vi "Software Update HCC Main Update HCC Software.vi"() -> ()   [LabVIEW 2016]
uses:
  Type Definitions/ViperHawk/ViperHawk Diagnostic Data.ctl
panel:
  in  "Update Files (Option 1-24)":i32[](array[numeric])
  in  "Tab Control 2":enum32{"Select Rows", "Find Active Stations"}(tab)
  out "% Complete":u8(slide) scale=0.0..100.0
  in  "Newfi":bool
  in  "Station 4":bool
  in  "Station 3":bool
  in  "Station 2":bool
  in  "Station 1":bool
  in  "Station 5":bool
  in  "Station 6":bool
  in  "Station 7":bool
  in  "Station 8":bool
  in  "Station 9":bool
  in  "Station 10":bool
  in  "Station 11":bool
  in  "Station 12":bool
  in  "Station 13":bool
  in  "Station 14":bool
  in  "Station 15":bool
  in  "Station 16":bool
  in  "Station 17":bool
  in  "Station 18":bool
  in  "Station 19":bool
  in  "Station 20":bool
  in  "Station 21":bool
  in  "Station 22":bool
  in  "Station 23":bool
  in  "Station 24":bool
  in  "Select All 1-4":bool caption="Select Row"
  in  "Select All 5-8":bool caption="Select Row"
  in  "Select All 9-12":bool caption="Select Row"
  in  "Select All 13-16":bool caption="Select Row"
  in  "Select All 17-20":bool caption="Select Row"
  in  "Select All 21-24":bool caption="Select Row"
  in  "Select All":bool
  out "Status String":string
  in  "New Software Location":path
  out "Debug Array":string[](array[string])
  in  "Debug":bool
  out "Main Directory":path
  in  "Find Active Stations":bool
  out "Active Stations with Board IDs":string[][](array[string])
  out "Board ID's":string[](array[string])
  out "Number of Newfi's":i32
  in  "Path Build List":path[](array[path])
  # "Software Update Tool"
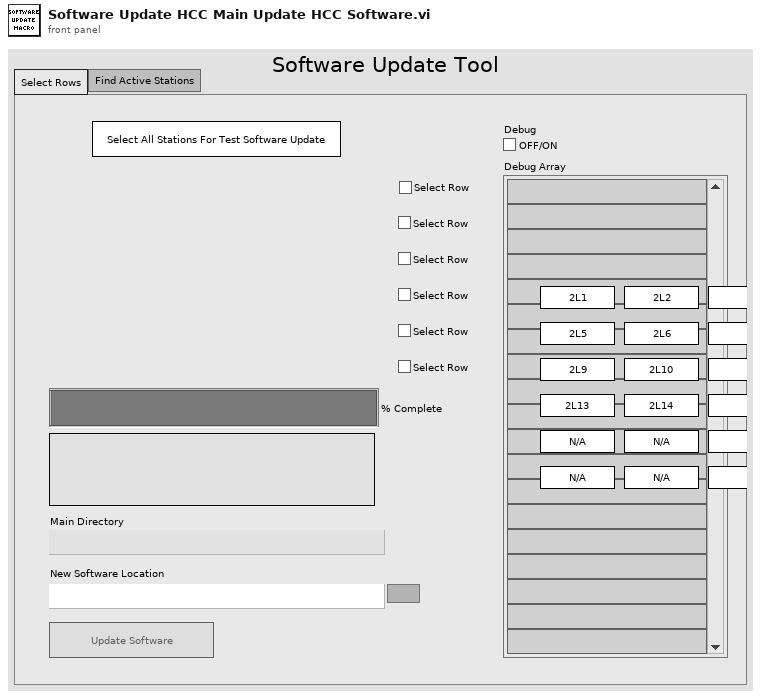
[diagram p1: front panel]
types:
  T1 = enum8{"Enabled", "Disabled", "Disabled and Grayed Out"}
  T2 = enum32{"invalid app kind", "Development System", "Run Time System", "Student Edition", "Embedded LabVIEW", "Evaluation", "Custom"}
  T3 = typedef "ViperHawk Diagnostic Data.ctl" = cluster{"Speed (RPM)":u32, "Load Size":u32, "Temperature":u32, "Water Pressure":dbl, "Detergent":u32, "Fabric Softener":u32, "Tub Direction":string, "Detergent Valve":bool, "Fabric Softener Valve":bool, "Recirculating Pump":bool, "Drain Valve":bool, "Hot Valve":bool, "Cold Valve":bool, "Lid Closed Status":string, "Lid Lock Status":string, "Error Count":u32, "IGBT Temperature (Deg C)":u32, "Motor Speed":u32, "Latched OOB":u32, "Raw OOB":u32, "Plaster Status":u32, "Inverter Power (W)":u32, "Target Speed(BRPM)":u32, "Latched Agitate Motor Temp (Deg C)":u32, "Current Motor Temp (Deg C)":u32, "Profiler Status":string, "Current Inverter Action":string, "Error Codes":string, "Lid Locked":bool, "Lid Closed":bool, "9E Diagnostic Data":cluster{"Total Cycle Time (Min)":u32, "Total Cycle Count (Current)":u16, "Total Error Count":u16, "Machine Error History":u32, "Washer UI History":u32, "Inverter Error History":u32, "Cycle Storage Limit":u8, "Error Storage Limit":u8, "Cycle Pages Supported":u8, "Error Pages Supported":u8, "Inverter Reset Count":u16}, "9F Diagnostic Data":cluster{"Cycle Buffer Index":string, "Page Number":string, "Total Cycle Count":u32, "Delay Start Time":u32, "Stain Selected":string, "Selected Cycle":u32, "eWash":string, "Soil Level":string, "Temperature":string, "Overnight Ready":string, "Spin Setting":string, "Control Lock Status":string, "Stain Remover":string, "Steam Assist":string, "My Cycle":string, "PreWash":string, "Debug Log Enabled":string, "Rinse":string, "Signal Level":string, "PreSoak":string}}
  T4 = enum32{"Invalid", "Standard", "Closed", "Hidden", "Minimized", "Maximized"}
  T5 = cluster{"Core":cluster{"Current VI Reference":refnum<vi>, "Close Panel on Exit?":bool}, "Base Newfi Exe Folder Path":path, "Path Build List":path[], "Update Files (Option 1-24)":i32[], "Diagnostic":T3}
  T6 = cluster{"Current VI Reference":refnum<vi>, "Close Panel on Exit?":bool}
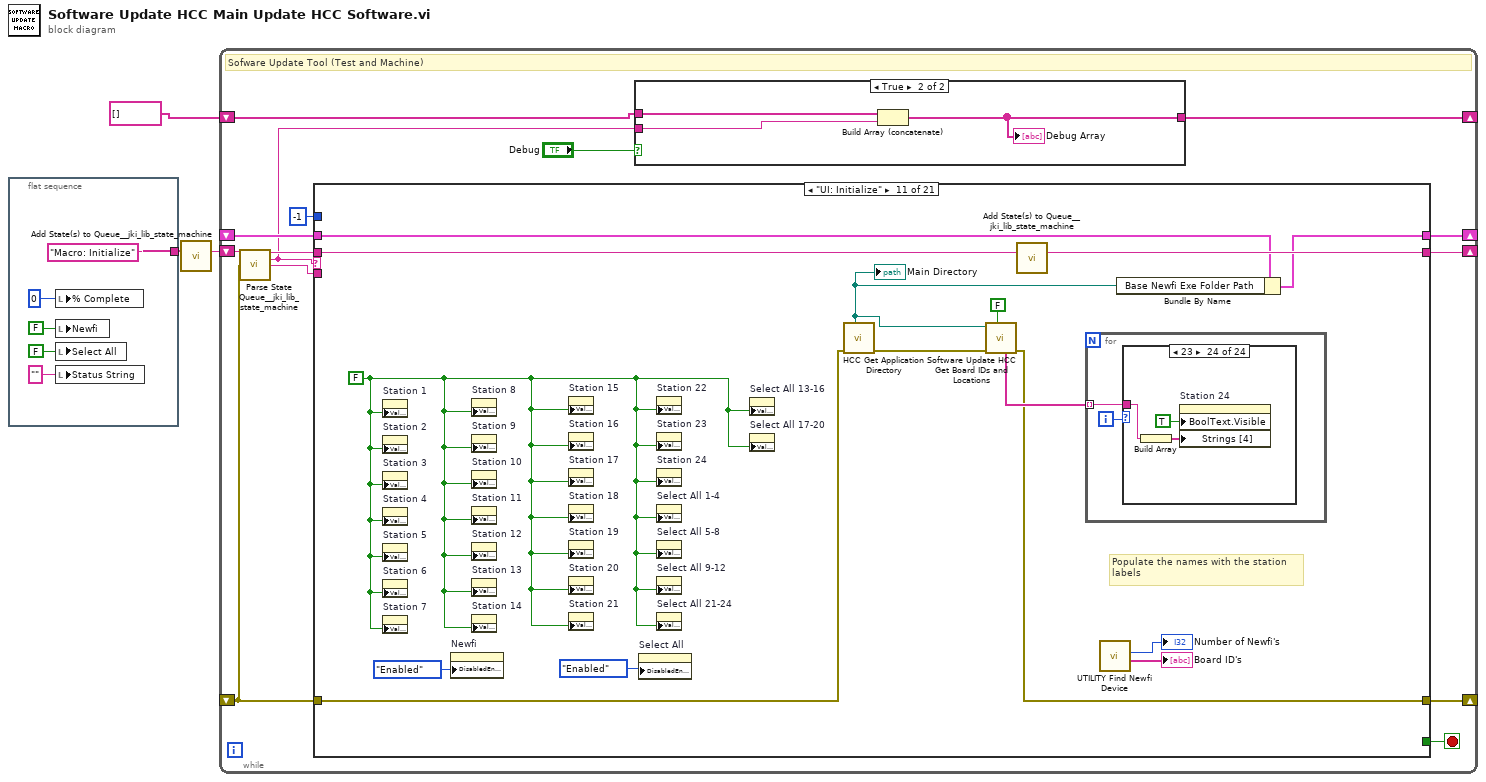
[diagram p0: block diagram]
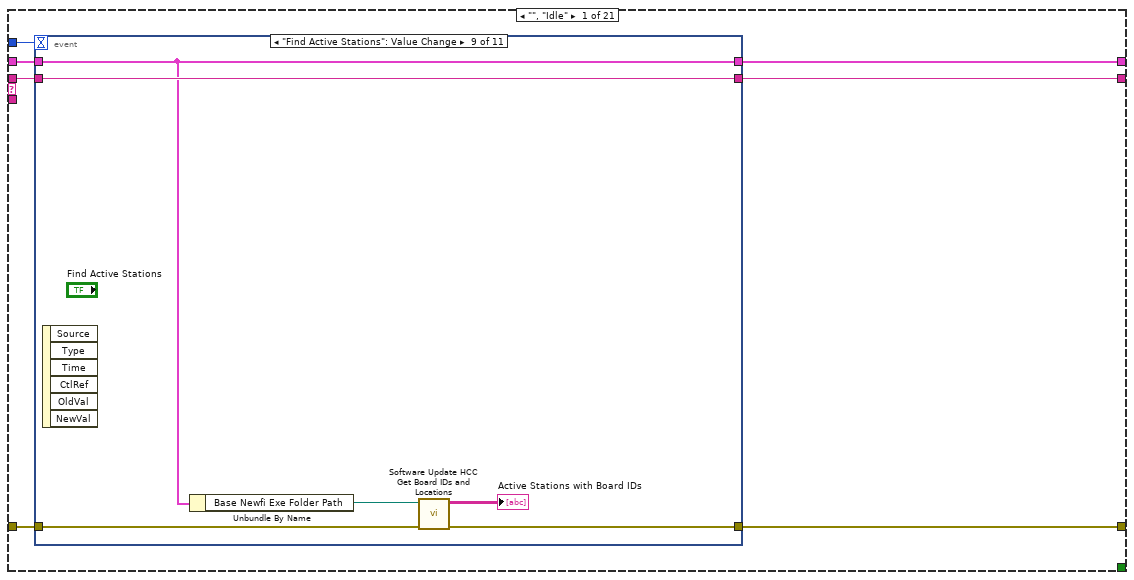
[diagram p3: hidden frame]
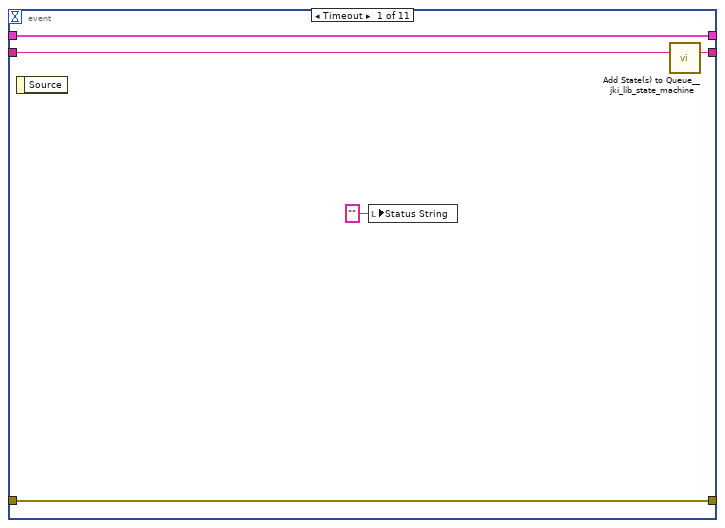
[diagram p4: hidden frame]
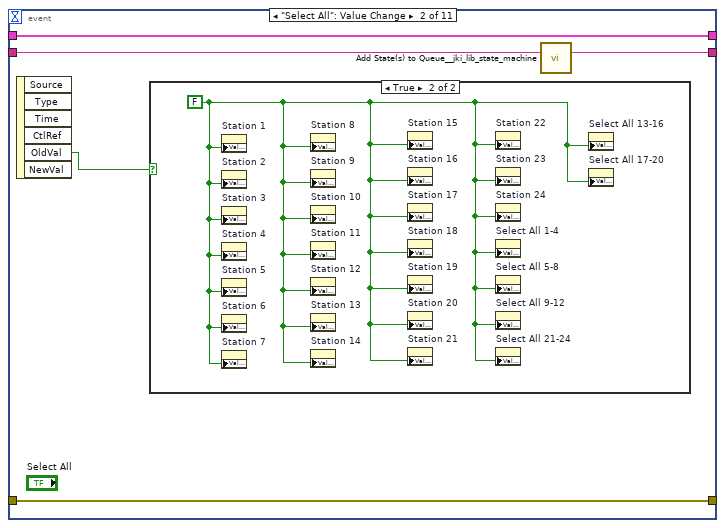
[diagram p5: hidden frame]
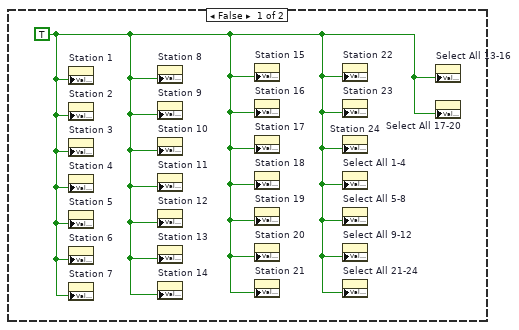
[diagram p6: hidden frame]
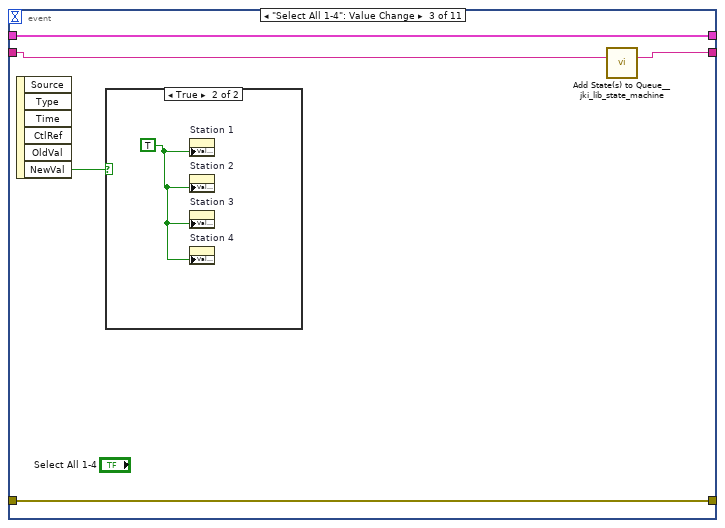
[diagram p7: hidden frame]
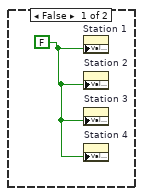
[diagram p8: hidden frame]
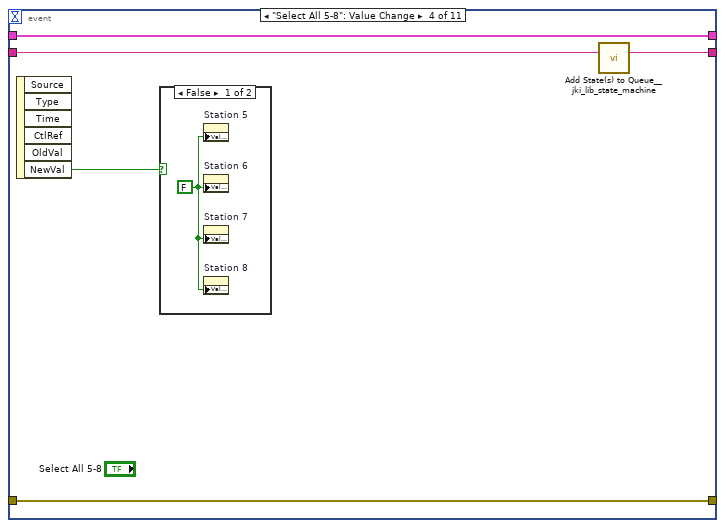
[diagram p9: hidden frame]
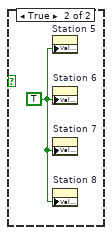
[diagram p10: hidden frame]
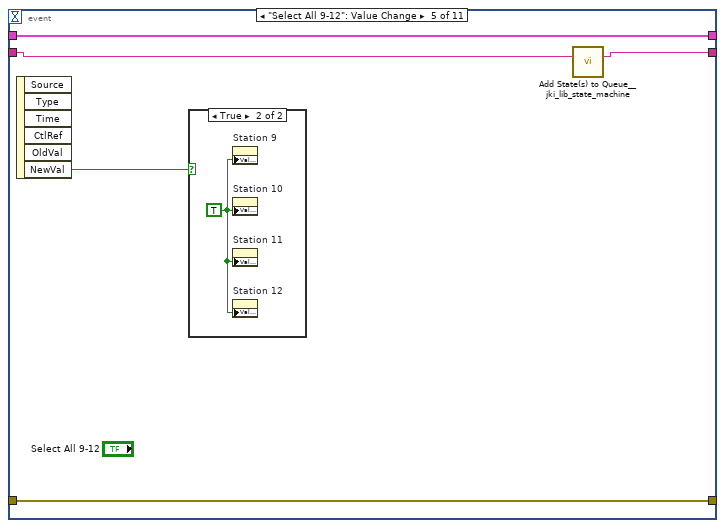
[diagram p11: hidden frame]
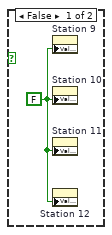
[diagram p12: hidden frame]
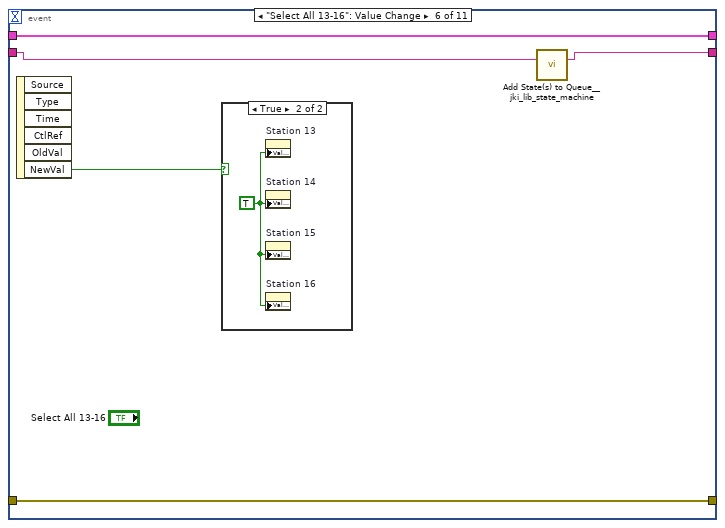
[diagram p13: hidden frame]
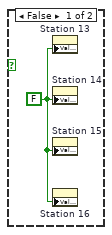
[diagram p14: hidden frame]
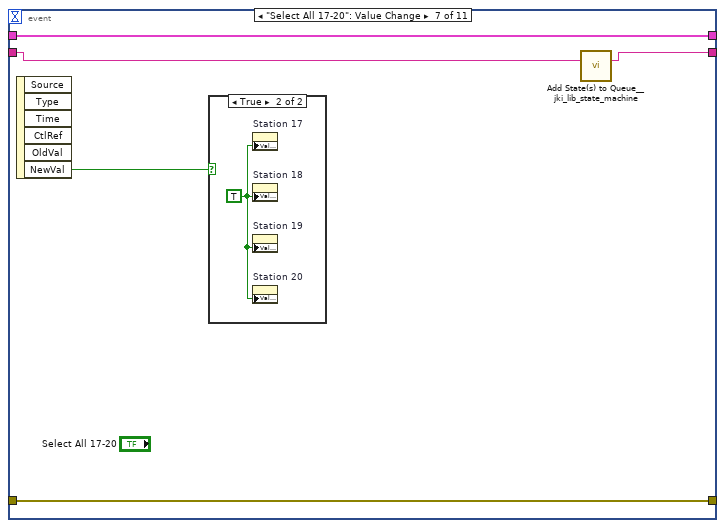
[diagram p15: hidden frame]
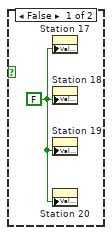
[diagram p16: hidden frame]
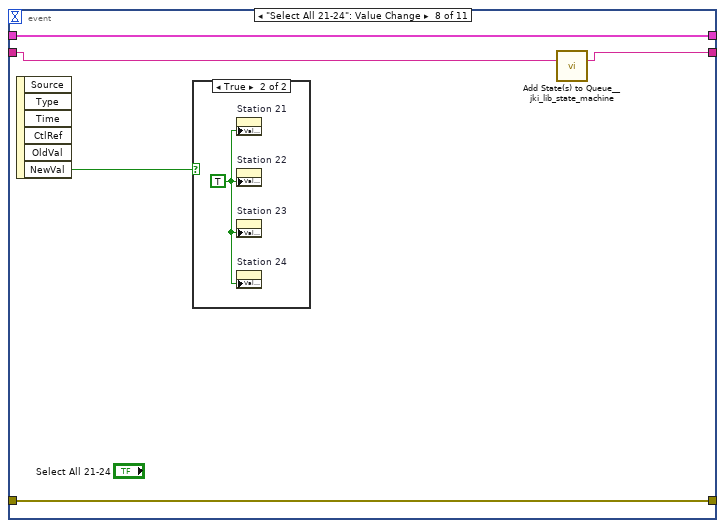
[diagram p17: hidden frame]
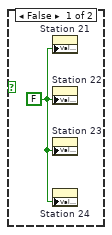
[diagram p18: hidden frame]
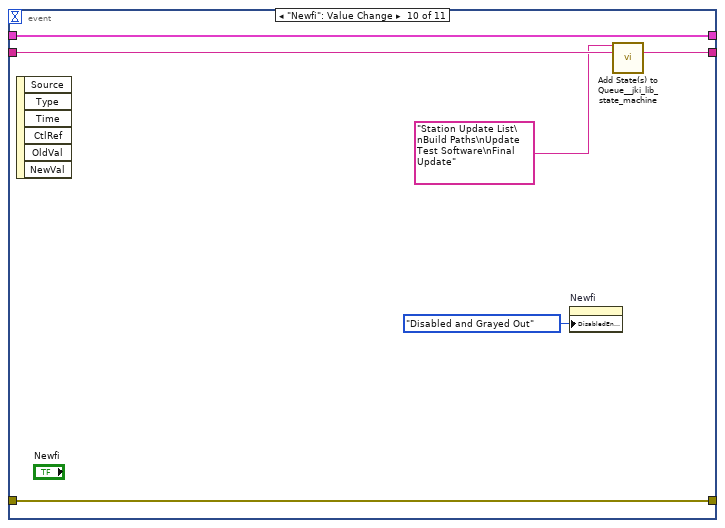
[diagram p19: hidden frame]
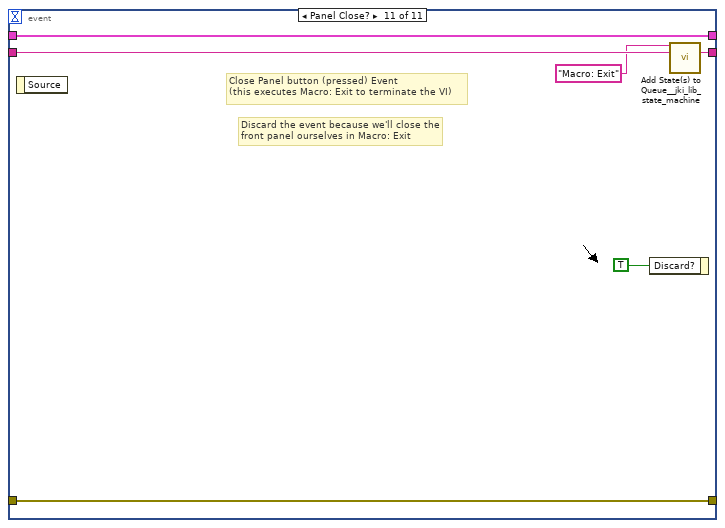
[diagram p20: hidden frame]
diagram:
  n1 = flat-sequence {
    tunnel: ["Macro: Initialize"] -> w2
    frame #0 {
      n2 = local write "% Complete"(u8 0 ("% Complete")) -> ()
      n3 = local write "Newfi"(FALSE ("Newfi")) -> ()
      n4 = local write "Select All"(FALSE ("Select All")) -> ()
      n5 = local write "Status String"("" ("Status String")) -> ()
    }
  }
  n6 = call <vilib>:"Add State(s) to Queue__jki_lib_state_machine.vi"("State(s) in (\"\")"=w2) -> ("States Out"=w3:string)  [unwired: 14 in]
  n7 = while "Sofware Update Tool (Test and Machine)" {
    shift-right: [w16] -> _
    shift-left: _ -> [w15]
    shift-right: [w19] -> _
    shift-left: _ -> [w13]
    shift-right: [w18] -> _
    shift-left: w3 -> [w20]
    shift-right: [w9] -> _
    shift-left: string[] [] -> [w12]
    stop <- w17 stop-if-true
    # "Sofware Update Tool (Test and Machine)"
    n8 = call <vilib>:"Parse State Queue__jki_lib_state_machine.vi"("State Queue"=w20, "Error In (no error)"=w13) -> ("Remaining States"=w22:string, "Current State"=w10:string, "Arguments"=w21:string)  [unwired: 11 in]
    n9 = case shown="\"UI: Initialize\"" w10 {
      selector: w10 -> [_ _ w110 _ _ _ _ _ _ _ _ _ _ _ _ _ _ _ _ _ _]
      tunnel: w22 -> [w33 w109 w114 w132 w138 w143 w147 w156 w162 w166 w181 w261 w272 w298 w303 w314 w318 w353 w363 w378 w386]
      tunnel: w21 -> [_ _ _ _ _ _ _ _ _ _ _ w256 w266 _ _ _ _ _ _ _ _]
      tunnel: w15 -> [w31 w106 w112 w123 w135 w141 w144 _ w157 w163 w169 w259 w268 w295 w300 w311 w315 w350 w360 w374 w384]
      tunnel: [w30 w107 w116 w129 errorcluster {"status"=FALSE, "code"=0, "source"=""} ("error out") w140 w145 w153 w158 w164 w170 w257 w269 w296 w301 w312 w316 w319 w356 w364 w383] -> w19
      tunnel: w13 -> [w29 w107 w115 w129 w134 w140 w145 w153 w159 w164 w171 w258 w270 w296 w301 w312 w316 w320 w357 w365 w383]
      tunnel: [w32 w108 w113 w131 w137 w142 w146 w155 w161 w165 w180 w260 w271 w297 w302 w313 w317 w352 w362 w377 w385] -> w18
      tunnel: [_ _ _ _ _ TRUE _ _ _ _ _ _ _ _ _ _ _ _ _ _ _] -> w17
      tunnel: [w28 w106 w112 w130 w135 w141 w144 w154 w157 w163 w168 w259 w268 w295 w300 w311 w315 w349 w359 w374 w384] -> w16
      tunnel: -1 ("Timeout") -> [w27 _ _ _ _ _ _ _ _ _ _ _ _ _ _ _ _ _ _ _ _]
      frame "", "Idle" {
        n10 = event shown="[8] \"Find Active Stations\": Value Change" {
          selector: _ -> [_ _ _ _ _ _ _ _ _ _ _]
          dyn-events: _ -> [_ _ _ _ _ _ _ _ _ _ _]
          timeout: w27 -> [_ _ _ _ _ _ _ _ _ _ _]
          tunnel: w33 -> [w38 w41 w48 w56 w63 w70 w77 w84 w90 w99 w105]
          tunnel: [w37 w40 w47 w55 w62 w69 w76 w83 w90 w98 w104] -> w32
          tunnel: w31 -> [w35 w43 w49 w57 w64 w71 w78 w85 w89 w94 w102]
          tunnel: [w36 w42 w50 w54 w61 w68 w75 w82 w91 w95 w103] -> w30
          tunnel: w29 -> [w36 w42 w50 w54 w61 w68 w75 w82 w92 w95 w103]
          tunnel: [w35 w43 w49 w57 w64 w71 w78 w85 w89 w94 w102] -> w28
          event Timeout {
            n11 = event-data() -> ()  [unwired: 1 in, 1 out]
            n12 = local write "Status String"("" ("Status String")) -> ()
            n13 = call <vilib>:"Add State(s) to Queue__jki_lib_state_machine.vi"("State(s) in (\"\")"=w38) -> ("States Out"=w37:string)  [unwired: 14 in]
          }
          event "Select All": Value Change {
            n14 = event-data() -> ("OldVal"=w39:bool)  [unwired: 1 in, 5 out]
            n15 = case shown="True" w39 {
              frame False {
                w44 = TRUE
                n16 = property on="Station 1" class="Bool (strict)"("Value"=w44) -> ()  [unwired: 2 in, 2 out]
                n17 = property on="Station 2" class="Bool (strict)"("Value"=w44) -> ()  [unwired: 2 in, 2 out]
                n18 = property on="Station 3" class="Bool (strict)"("Value"=w44) -> ()  [unwired: 2 in, 2 out]
                n19 = property on="Station 4" class="Bool (strict)"("Value"=w44) -> ()  [unwired: 2 in, 2 out]
                n20 = property on="Station 5" class="Bool (strict)"("Value"=w44) -> ()  [unwired: 2 in, 2 out]
                n21 = property on="Station 6" class="Bool (strict)"("Value"=w44) -> ()  [unwired: 2 in, 2 out]
                n22 = property on="Station 7" class="Bool (strict)"("Value"=w44) -> ()  [unwired: 2 in, 2 out]
                n23 = property on="Station 8" class="Bool (strict)"("Value"=w44) -> ()  [unwired: 2 in, 2 out]
                n24 = property on="Station 9" class="Bool (strict)"("Value"=w44) -> ()  [unwired: 2 in, 2 out]
                n25 = property on="Station 10" class="Bool (strict)"("Value"=w44) -> ()  [unwired: 2 in, 2 out]
                n26 = property on="Station 11" class="Bool (strict)"("Value"=w44) -> ()  [unwired: 2 in, 2 out]
                n27 = property on="Station 12" class="Bool (strict)"("Value"=w44) -> ()  [unwired: 2 in, 2 out]
                n28 = property on="Station 13" class="Bool (strict)"("Value"=w44) -> ()  [unwired: 2 in, 2 out]
                n29 = property on="Station 14" class="Bool (strict)"("Value"=w44) -> ()  [unwired: 2 in, 2 out]
                n30 = property on="Station 15" class="Bool (strict)"("Value"=w44) -> ()  [unwired: 2 in, 2 out]
                n31 = property on="Station 16" class="Bool (strict)"("Value"=w44) -> ()  [unwired: 2 in, 2 out]
                n32 = property on="Station 17" class="Bool (strict)"("Value"=w44) -> ()  [unwired: 2 in, 2 out]
                n33 = property on="Station 18" class="Bool (strict)"("Value"=w44) -> ()  [unwired: 2 in, 2 out]
                n34 = property on="Station 19" class="Bool (strict)"("Value"=w44) -> ()  [unwired: 2 in, 2 out]
                n35 = property on="Station 20" class="Bool (strict)"("Value"=w44) -> ()  [unwired: 2 in, 2 out]
                n36 = property on="Station 21" class="Bool (strict)"("Value"=w44) -> ()  [unwired: 2 in, 2 out]
                n37 = property on="Station 22" class="Bool (strict)"("Value"=w44) -> ()  [unwired: 2 in, 2 out]
                n38 = property on="Station 23" class="Bool (strict)"("Value"=w44) -> ()  [unwired: 2 in, 2 out]
                n39 = property on="Station 24" class="Bool (strict)"("Value"=w44) -> ()  [unwired: 2 in, 2 out]
                n40 = property on="Select All 1-4" class="Bool (strict)"("Value"=w44) -> ()  [unwired: 2 in, 2 out]
                n41 = property on="Select All 5-8" class="Bool (strict)"("Value"=w44) -> ()  [unwired: 2 in, 2 out]
                n42 = property on="Select All 9-12" class="Bool (strict)"("Value"=w44) -> ()  [unwired: 2 in, 2 out]
                n43 = property on="Select All 21-24" class="Bool (strict)"("Value"=w44) -> ()  [unwired: 2 in, 2 out]
                n44 = property on="Select All 13-16" class="Bool (strict)"("Value"=w44) -> ()  [unwired: 2 in, 2 out]
                n45 = property on="Select All 17-20" class="Bool (strict)"("Value"=w44) -> ()  [unwired: 2 in, 2 out]
              }
              frame True {
                w45 = FALSE
                n46 = property on="Station 1" class="Bool (strict)"("Value"=w45) -> ()  [unwired: 2 in, 2 out]
                n47 = property on="Station 2" class="Bool (strict)"("Value"=w45) -> ()  [unwired: 2 in, 2 out]
                n48 = property on="Station 3" class="Bool (strict)"("Value"=w45) -> ()  [unwired: 2 in, 2 out]
                n49 = property on="Station 4" class="Bool (strict)"("Value"=w45) -> ()  [unwired: 2 in, 2 out]
                n50 = property on="Station 5" class="Bool (strict)"("Value"=w45) -> ()  [unwired: 2 in, 2 out]
                n51 = property on="Station 6" class="Bool (strict)"("Value"=w45) -> ()  [unwired: 2 in, 2 out]
                n52 = property on="Station 7" class="Bool (strict)"("Value"=w45) -> ()  [unwired: 2 in, 2 out]
                n53 = property on="Station 8" class="Bool (strict)"("Value"=w45) -> ()  [unwired: 2 in, 2 out]
                n54 = property on="Station 9" class="Bool (strict)"("Value"=w45) -> ()  [unwired: 2 in, 2 out]
                n55 = property on="Station 10" class="Bool (strict)"("Value"=w45) -> ()  [unwired: 2 in, 2 out]
                n56 = property on="Station 11" class="Bool (strict)"("Value"=w45) -> ()  [unwired: 2 in, 2 out]
                n57 = property on="Station 12" class="Bool (strict)"("Value"=w45) -> ()  [unwired: 2 in, 2 out]
                n58 = property on="Station 13" class="Bool (strict)"("Value"=w45) -> ()  [unwired: 2 in, 2 out]
                n59 = property on="Station 14" class="Bool (strict)"("Value"=w45) -> ()  [unwired: 2 in, 2 out]
                n60 = property on="Station 15" class="Bool (strict)"("Value"=w45) -> ()  [unwired: 2 in, 2 out]
                n61 = property on="Station 16" class="Bool (strict)"("Value"=w45) -> ()  [unwired: 2 in, 2 out]
                n62 = property on="Station 17" class="Bool (strict)"("Value"=w45) -> ()  [unwired: 2 in, 2 out]
                n63 = property on="Station 18" class="Bool (strict)"("Value"=w45) -> ()  [unwired: 2 in, 2 out]
                n64 = property on="Station 19" class="Bool (strict)"("Value"=w45) -> ()  [unwired: 2 in, 2 out]
                n65 = property on="Station 20" class="Bool (strict)"("Value"=w45) -> ()  [unwired: 2 in, 2 out]
                n66 = property on="Station 21" class="Bool (strict)"("Value"=w45) -> ()  [unwired: 2 in, 2 out]
                n67 = property on="Station 22" class="Bool (strict)"("Value"=w45) -> ()  [unwired: 2 in, 2 out]
                n68 = property on="Station 23" class="Bool (strict)"("Value"=w45) -> ()  [unwired: 2 in, 2 out]
                n69 = property on="Station 24" class="Bool (strict)"("Value"=w45) -> ()  [unwired: 2 in, 2 out]
                n70 = property on="Select All 1-4" class="Bool (strict)"("Value"=w45) -> ()  [unwired: 2 in, 2 out]
                n71 = property on="Select All 5-8" class="Bool (strict)"("Value"=w45) -> ()  [unwired: 2 in, 2 out]
                n72 = property on="Select All 9-12" class="Bool (strict)"("Value"=w45) -> ()  [unwired: 2 in, 2 out]
                n73 = property on="Select All 21-24" class="Bool (strict)"("Value"=w45) -> ()  [unwired: 2 in, 2 out]
                n74 = property on="Select All 13-16" class="Bool (strict)"("Value"=w45) -> ()  [unwired: 2 in, 2 out]
                n75 = property on="Select All 17-20" class="Bool (strict)"("Value"=w45) -> ()  [unwired: 2 in, 2 out]
              }
            }
            n76 = call <vilib>:"Add State(s) to Queue__jki_lib_state_machine.vi"("State(s) in (\"\")"=w41) -> ("States Out"=w40:string)  [unwired: 14 in]
          }
          event "Select All 1-4": Value Change {
            n77 = event-data() -> ("NewVal"=w46:bool)  [unwired: 1 in, 5 out]
            n78 = case shown="True" w46 {
              frame False {
                w51 = FALSE
                n79 = property on="Station 1" class="Bool (strict)"("Value"=w51) -> ()  [unwired: 2 in, 2 out]
                n80 = property on="Station 2" class="Bool (strict)"("Value"=w51) -> ()  [unwired: 2 in, 2 out]
                n81 = property on="Station 3" class="Bool (strict)"("Value"=w51) -> ()  [unwired: 2 in, 2 out]
                n82 = property on="Station 4" class="Bool (strict)"("Value"=w51) -> ()  [unwired: 2 in, 2 out]
              }
              frame True {
                w52 = TRUE
                n83 = property on="Station 1" class="Bool (strict)"("Value"=w52) -> ()  [unwired: 2 in, 2 out]
                n84 = property on="Station 2" class="Bool (strict)"("Value"=w52) -> ()  [unwired: 2 in, 2 out]
                n85 = property on="Station 3" class="Bool (strict)"("Value"=w52) -> ()  [unwired: 2 in, 2 out]
                n86 = property on="Station 4" class="Bool (strict)"("Value"=w52) -> ()  [unwired: 2 in, 2 out]
              }
            }
            n87 = call <vilib>:"Add State(s) to Queue__jki_lib_state_machine.vi"("State(s) in (\"\")"=w48) -> ("States Out"=w47:string)  [unwired: 14 in]
          }
          event "Select All 5-8": Value Change {
            n88 = event-data() -> ("NewVal"=w53:bool)  [unwired: 1 in, 5 out]
            n89 = case shown="False" w53 {
              frame False {
                w58 = FALSE ("Visible")
                n90 = property on="Station 5" class="Bool (strict)"("Value"=w58) -> ()  [unwired: 2 in, 2 out]
                n91 = property on="Station 6" class="Bool (strict)"("Value"=w58) -> ()  [unwired: 2 in, 2 out]
                n92 = property on="Station 7" class="Bool (strict)"("Value"=w58) -> ()  [unwired: 2 in, 2 out]
                n93 = property on="Station 8" class="Bool (strict)"("Value"=w58) -> ()  [unwired: 2 in, 2 out]
              }
              frame True {
                w59 = TRUE ("Visible")
                n94 = property on="Station 5" class="Bool (strict)"("Value"=w59) -> ()  [unwired: 2 in, 2 out]
                n95 = property on="Station 6" class="Bool (strict)"("Value"=w59) -> ()  [unwired: 2 in, 2 out]
                n96 = property on="Station 7" class="Bool (strict)"("Value"=w59) -> ()  [unwired: 2 in, 2 out]
                n97 = property on="Station 8" class="Bool (strict)"("Value"=w59) -> ()  [unwired: 2 in, 2 out]
              }
            }
            n98 = call <vilib>:"Add State(s) to Queue__jki_lib_state_machine.vi"("State(s) in (\"\")"=w56) -> ("States Out"=w55:string)  [unwired: 14 in]
          }
          event "Select All 9-12": Value Change {
            n99 = event-data() -> ("NewVal"=w60:bool)  [unwired: 1 in, 5 out]
            n100 = case shown="True" w60 {
              frame False {
                w65 = FALSE
                n101 = property on="Station 9" class="Bool (strict)"("Value"=w65) -> ()  [unwired: 2 in, 2 out]
                n102 = property on="Station 10" class="Bool (strict)"("Value"=w65) -> ()  [unwired: 2 in, 2 out]
                n103 = property on="Station 11" class="Bool (strict)"("Value"=w65) -> ()  [unwired: 2 in, 2 out]
                n104 = property on="Station 12" class="Bool (strict)"("Value"=w65) -> ()  [unwired: 2 in, 2 out]
              }
              frame True {
                w66 = TRUE ("Visible")
                n105 = property on="Station 9" class="Bool (strict)"("Value"=w66) -> ()  [unwired: 2 in, 2 out]
                n106 = property on="Station 10" class="Bool (strict)"("Value"=w66) -> ()  [unwired: 2 in, 2 out]
                n107 = property on="Station 11" class="Bool (strict)"("Value"=w66) -> ()  [unwired: 2 in, 2 out]
                n108 = property on="Station 12" class="Bool (strict)"("Value"=w66) -> ()  [unwired: 2 in, 2 out]
              }
            }
            n109 = call <vilib>:"Add State(s) to Queue__jki_lib_state_machine.vi"("State(s) in (\"\")"=w63) -> ("States Out"=w62:string)  [unwired: 14 in]
          }
          event "Select All 13-16": Value Change {
            n110 = event-data() -> ("NewVal"=w67:bool)  [unwired: 1 in, 5 out]
            n111 = case shown="True" w67 {
              frame False {
                w72 = FALSE
                n112 = property on="Station 13" class="Bool (strict)"("Value"=w72) -> ()  [unwired: 2 in, 2 out]
                n113 = property on="Station 14" class="Bool (strict)"("Value"=w72) -> ()  [unwired: 2 in, 2 out]
                n114 = property on="Station 15" class="Bool (strict)"("Value"=w72) -> ()  [unwired: 2 in, 2 out]
                n115 = property on="Station 16" class="Bool (strict)"("Value"=w72) -> ()  [unwired: 2 in, 2 out]
              }
              frame True {
                w73 = TRUE
                n116 = property on="Station 13" class="Bool (strict)"("Value"=w73) -> ()  [unwired: 2 in, 2 out]
                n117 = property on="Station 14" class="Bool (strict)"("Value"=w73) -> ()  [unwired: 2 in, 2 out]
                n118 = property on="Station 15" class="Bool (strict)"("Value"=w73) -> ()  [unwired: 2 in, 2 out]
                n119 = property on="Station 16" class="Bool (strict)"("Value"=w73) -> ()  [unwired: 2 in, 2 out]
              }
            }
            n120 = call <vilib>:"Add State(s) to Queue__jki_lib_state_machine.vi"("State(s) in (\"\")"=w70) -> ("States Out"=w69:string)  [unwired: 14 in]
          }
          event "Select All 17-20": Value Change {
            n121 = event-data() -> ("NewVal"=w74:bool)  [unwired: 1 in, 5 out]
            n122 = case shown="True" w74 {
              frame False {
                w79 = FALSE
                n123 = property on="Station 17" class="Bool (strict)"("Value"=w79) -> ()  [unwired: 2 in, 2 out]
                n124 = property on="Station 18" class="Bool (strict)"("Value"=w79) -> ()  [unwired: 2 in, 2 out]
                n125 = property on="Station 19" class="Bool (strict)"("Value"=w79) -> ()  [unwired: 2 in, 2 out]
                n126 = property on="Station 20" class="Bool (strict)"("Value"=w79) -> ()  [unwired: 2 in, 2 out]
              }
              frame True {
                w80 = TRUE
                n127 = property on="Station 17" class="Bool (strict)"("Value"=w80) -> ()  [unwired: 2 in, 2 out]
                n128 = property on="Station 18" class="Bool (strict)"("Value"=w80) -> ()  [unwired: 2 in, 2 out]
                n129 = property on="Station 19" class="Bool (strict)"("Value"=w80) -> ()  [unwired: 2 in, 2 out]
                n130 = property on="Station 20" class="Bool (strict)"("Value"=w80) -> ()  [unwired: 2 in, 2 out]
              }
            }
            n131 = call <vilib>:"Add State(s) to Queue__jki_lib_state_machine.vi"("State(s) in (\"\")"=w77) -> ("States Out"=w76:string)  [unwired: 14 in]
          }
          event "Select All 21-24": Value Change {
            n132 = event-data() -> ("NewVal"=w81:bool)  [unwired: 1 in, 5 out]
            n133 = case shown="True" w81 {
              frame False {
                w86 = FALSE
                n134 = property on="Station 21" class="Bool (strict)"("Value"=w86) -> ()  [unwired: 2 in, 2 out]
                n135 = property on="Station 22" class="Bool (strict)"("Value"=w86) -> ()  [unwired: 2 in, 2 out]
                n136 = property on="Station 23" class="Bool (strict)"("Value"=w86) -> ()  [unwired: 2 in, 2 out]
                n137 = property on="Station 24" class="Bool (strict)"("Value"=w86) -> ()  [unwired: 2 in, 2 out]
              }
              frame True {
                w87 = TRUE
                n138 = property on="Station 21" class="Bool (strict)"("Value"=w87) -> ()  [unwired: 2 in, 2 out]
                n139 = property on="Station 22" class="Bool (strict)"("Value"=w87) -> ()  [unwired: 2 in, 2 out]
                n140 = property on="Station 23" class="Bool (strict)"("Value"=w87) -> ()  [unwired: 2 in, 2 out]
                n141 = property on="Station 24" class="Bool (strict)"("Value"=w87) -> ()  [unwired: 2 in, 2 out]
              }
            }
            n142 = call <vilib>:"Add State(s) to Queue__jki_lib_state_machine.vi"("State(s) in (\"\")"=w84) -> ("States Out"=w83:string)  [unwired: 14 in]
          }
          event "Find Active Stations": Value Change {
            n143 = event-data() -> ()  [unwired: 1 in, 6 out]
            n144 = Unbundle By Name(w89) -> ("Base Newfi Exe Folder Path"=w88:path)
            n145 = call "Software Update HCC Get Board IDs and Locations.vi"("Error In"=w92, "Newfi Exe Folder Path"=w88) -> ("Error Out"=w91:errorcluster, "Active Stations with Board IDs"=→"Active Stations with Board IDs":string[][])  [unwired: 6 in, 2 out]
          }
          event "Newfi": Value Change {
            n146 = event-data() -> ()  [unwired: 1 in, 6 out]
            n147 = property on="Newfi" class="Bool (strict)"("DisabledEnum"=T1."Disabled and Grayed Out" ("Disabled")) -> ()  [unwired: 2 in, 2 out]
            n148 = call <vilib>:"Add State(s) to Queue__jki_lib_state_machine.vi"("State(s) in Front (\"\")"="Station Update List\nBuild Paths\nUpdate Test Software\nFinal Update", "State(s) in (\"\")"=w99) -> ("States Out"=w98:string)  [unwired: 13 in]
          }
          event Panel Close? {
            # "Discard the event because we'll close the front panel ourselves in Macro: Exit"
            # "Close Panel button (pressed) Event\n(this executes Macro: Exit to terminate the VI)"
            n149 = event-data() -> ()  [unwired: 1 in, 1 out]
            n150 = event-data("Discard?"=TRUE) -> ()  [unwired: 1 in, 1 out]
            n151 = call <vilib>:"Add State(s) to Queue__jki_lib_state_machine.vi"("State(s) in Front (\"\")"="Macro: Exit", "State(s) in (\"\")"=w105) -> ("States Out"=w104:string)  [unwired: 13 in]
          }
        }
      }
      frame "---------- Core ----------" {
        # "Do not put any code in this frame.\n(it is a separator no-op)"
        n152 = call <vilib>:"Add State(s) to Queue__jki_lib_state_machine.vi"("State(s) in (\"\")"=w109) -> ("States Out"=w108:string)  [unwired: 14 in]
      }
      frame Default {
        w119 = 42 items=["No error", "Argument error", "Memory is full", "Out of zone", "End of file", "File already open", "Generic file I/O error", "File not found", "File permission error", "Disk is full", "Duplicate path", "Too many files open", "System feature not enabled", "Resource file not found", "Cannot add resource", "Resource not found", "Image not found", "Image memory error", "Pen does not exist", "Config type invalid", "Config token not found", "Config parse error", "Config memory error", "Bad external code format", "Bad external code offset", "External code not present", "Null window", "Destroy window error", "Null menu", "Print aborted", "Bad print record", "Print driver error", "Windows error during printing", "Memory error during printing", "Print dialog error", "Generic print error", "Invalid device refnum", "Device not found", "Device parameter error", "Device unit error", "Cannot open device", "Device call aborted", "Generic error", "Cancelled by user", "Object ID too low", "Object ID too high", "Object not in heap", "Unknown heap", "Unknown object (invalid DefProc)", "Unknown object (DefProc not in table)", "Message out of range", "Invalid (null) method", "Unknown message", "Manager call not supported", "Bad address", "Network operation in progress", "Network operation timed out", "Connection is busy", "Network attribute not supported", "Network error", "Address in use", "System out of memory", "Connection aborted", "Connection refused", "Not connected", "Already connected", "Connection closed", "Initialization error (interapplication manager)", "Bad occurrence", "Wait on unbound occurrence handler", "Occurrence queue overflow", "Datalog type conflict", "Unused", "Unrecognized type (interapplication manager)", "Memory corrupt", "Failed to make temporary DLL", "Old CIN version", "Drag socket not found", "Failed to load drop-object", "Failed to register OLE object", "Failed to release OLE object", "Format specifier type mismatch", "Unknown format specifier", "Too few format specifiers", "Too many format specifiers", "Scan failed", "Newer CIN version", "Error converting to variant", "Runtime menu error", "Password tampered", "Variant attribute not found", "Incompatible variant data type", "Event data is not available", "Event Store is not present", "Occurrence is not found", "Event Queue is not created", "Event info is not available", "Refnum passed is NULL", "Error retrieving Class GUID", "Error retrieving CoClass GUID", "Error retrieving TypeLib GUID.", "Bad built application magic bytes.", "Specific driver is different from the specific driver associated with the Logical Name.", "There is no session opened to the class driver.", "Max Error", "MAX - Error with config objects", "MAX - Error loading configuration", "MAX - Group not supported"]
        # "Current State"
        # "Do not delete, rename, or modify this frame.\n(this is used to capture unhandled states and typos)"
        # "Handle mistyped state name (developer tool)"
        n153 = Format Into String(format string="Software Exception: Unhandled State \"%s\"." ("message"), error in=w115, w110) -> (resulting string=w118:string, error out=w117:errorcluster)  [unwired: 1 in]
        n154 = call <vilib>:"Error Cluster From Error Code.vi"("show call chain? (False)"=TRUE, "error in (no error)"=w117, "error message (\"\")"=w118, "error code (0)"=w119) -> ("error out"=w116:errorcluster)  [unwired: 5 in]
        n155 = call <vilib>:"Add State(s) to Queue__jki_lib_state_machine.vi"("State(s) in (\"\")"=w114) -> ("States Out"=w113:string)  [unwired: 14 in]
      }
      frame "Initialize Core Data" {
        # "Do not delete, rename, or modify this frame.\n(this is used to determine panel behavior on exit)"
        # "originally closed?"
        # "exe?"
        # "If panel starts closed or is an EXE, then close it when we exit"
        n156 = property class="VI"() -> ("Front Panel.Open"=w128:bool)  [unwired: 2 in, 2 out]
        n157 = property class="App"() -> ("App.Kind"=w127:T2)  [unwired: 2 in, 2 out]
        n158 = control-ref of="Current VI Reference"() -> (w121:refnum<vi>)
        n159 = Not(x=w128) -> (.not. x?=w125:bool)
        n160 = Equal?(x=w127, y=T2."Run Time System" ("Application:Kind")) -> (x = y?=w124:bool)
        n161 = Or(x=w125, y=w124) -> (x .or. y?=w122:bool)
        n162 = Bundle By Name(cluster=w123, "Core.Current VI Reference"=w121, "Core.Close Panel on Exit?"=w122) -> (w130:T5)
        n163 = call <vilib>:"Add State(s) to Queue__jki_lib_state_machine.vi"("State(s) in (\"\")"=w132) -> ("States Out"=w131:string)  [unwired: 14 in]
      }
      frame "Error Handler" {
        # "Unhandled Error -- Display it"
        # "Handle any errors here.\nYou can also output any states to clean-up after errors occur"
        # "Clear error"
        n164 = call <vilib>:"General Error Handler.vi"("error in (no error)"=w134) -> ()  [unwired: 10 in, 5 out]
        n165 = call <vilib>:"Add State(s) to Queue__jki_lib_state_machine.vi"("State(s) in Front (\"\")"="/* Post Error States", "State(s) in (\"\")"=w138) -> ("States Out"=w137:string)  [unwired: 13 in]
      }
      frame "Exit" {
        # "Do not put any code in this frame.\n(No errors that occur here will be handled.)"
        n166 = call <vilib>:"Add State(s) to Queue__jki_lib_state_machine.vi"("State(s) in (\"\")"=w143) -> ("States Out"=w142:string)  [unwired: 14 in]
      }
      frame "---------- Data ----------" {
        # "Do not put any code in this frame.\n(It is a separator no-op. You can make a copy of this frame to create a new Data frame)"
        n167 = call <vilib>:"Add State(s) to Queue__jki_lib_state_machine.vi"("State(s) in (\"\")"=w147) -> ("States Out"=w146:string)  [unwired: 14 in]
      }
      frame "Data: Initialize" {
        w152 = T6 {"Current VI Reference"=refnum, "Close Panel on Exit?"=FALSE}  # Core
        n168 = Bundle("Core"=w152, "Base Newfi Exe Folder Path"=path "", "Path Build List"="Path Build List", "Update Files (Option 1-24)"="Update Files (Option 1-24)", "Diagnostic"=T3 {"Speed (RPM)"=0, "Load Size"=0, "Temperature"=0, "Water Pressure"=0.0, "Detergent"=0, "Fabric Softener"=0, "Tub Direction"="", "Detergent Valve"=FALSE, "Fabric Softener Valve"=FALSE, "Recirculating Pump"=FALSE, "Drain Valve"=FALSE, "Hot Valve"=FALSE, "Cold Valve"=FALSE, "Lid Closed Status"="", "Lid Lock Status"="", "Error Count"=0, "IGBT Temperature (Deg C)"=0, "Motor Speed"=0, "Latched OOB"=0, "Raw OOB"=0, "Plaster Status"=0, "Inverter Power (W)"=0, "Target Speed(BRPM)"=0, "Latched Agitate Motor Temp (Deg C)"=0, "Current Motor Temp (Deg C)"=0, "Profiler Status"="", "Current Inverter Action"="", "Error Codes"="", "Lid Locked"=FALSE, "Lid Closed"=FALSE, "9E Diagnostic Data"={"Total Cycle Time (Min)"=0, "Total Cycle Count (Current)"=0, "Total Error Count"=0, "Machine Error History"=0, "Washer UI History"=0, "Inverter Error History"=0, "Cycle Storage Limit"=0, "Error Storage Limit"=0, "Cycle Pages Supported"=0, "Error Pages Supported"=0, "Inverter Reset Count"=0}, "9F Diagnostic Data"={"Cycle Buffer Index"="", "Page Number"="", "Total Cycle Count"=0, "Delay Start Time"=0, "Stain Selected"="", "Selected Cycle"=0, "eWash"="", "Soil Level"="", "Temperature"="", "Overnight Ready"="", "Spin Setting"="", "Control Lock Status"="", "Stain Remover"="", "Steam Assist"="", "My Cycle"="", "PreWash"="", "Debug Log Enabled"="", "Rinse"="", "Signal Level"="", "PreSoak"=""}}) -> (w154:T5)  [unwired: 1 in]
        n169 = call <vilib>:"Add State(s) to Queue__jki_lib_state_machine.vi"("State(s) in (\"\")"=w156) -> ("States Out"=w155:string)  [unwired: 14 in]
      }
      frame "Data: Cleanup" {
        # "Cleanup any data and references, here.\n(this is called automatically, by the Macro: Exit)"
        n170 = Unbundle By Name(w157) -> ("Core.Current VI Reference"=w160:refnum<vi>)
        n171 = Close Reference(reference=w160, error in (no error)=w159) -> (error out=w158:errorcluster)
        n172 = call <vilib>:"Add State(s) to Queue__jki_lib_state_machine.vi"("State(s) in (\"\")"=w162) -> ("States Out"=w161:string)  [unwired: 14 in]
      }
      frame "---------- UI ----------" {
        # "Do not put any code in this frame.\n(It is a separator no-op. You can make a copy of this frame to create a new UI frame)"
        n173 = call <vilib>:"Add State(s) to Queue__jki_lib_state_machine.vi"("State(s) in (\"\")"=w166) -> ("States Out"=w165:string)  [unwired: 14 in]
      }
      frame "UI: Initialize" {
        w176 = FALSE
        # "Populate the names with the station\nlabels"
        n174 = property on="Station 1" class="Bool (strict)"("Value"=w176) -> ()  [unwired: 2 in, 2 out]
        n175 = property on="Station 2" class="Bool (strict)"("Value"=w176) -> ()  [unwired: 2 in, 2 out]
        n176 = property on="Station 3" class="Bool (strict)"("Value"=w176) -> ()  [unwired: 2 in, 2 out]
        n177 = property on="Station 4" class="Bool (strict)"("Value"=w176) -> ()  [unwired: 2 in, 2 out]
        n178 = property on="Station 5" class="Bool (strict)"("Value"=w176) -> ()  [unwired: 2 in, 2 out]
        n179 = property on="Station 6" class="Bool (strict)"("Value"=w176) -> ()  [unwired: 2 in, 2 out]
        n180 = property on="Station 7" class="Bool (strict)"("Value"=w176) -> ()  [unwired: 2 in, 2 out]
        n181 = property on="Newfi" class="Bool (strict)"("DisabledEnum"=T1."Enabled" ("Disabled")) -> ()  [unwired: 2 in, 2 out]
        n182 = property on="Station 8" class="Bool (strict)"("Value"=w176) -> ()  [unwired: 2 in, 2 out]
        n183 = property on="Station 9" class="Bool (strict)"("Value"=w176) -> ()  [unwired: 2 in, 2 out]
        n184 = property on="Station 10" class="Bool (strict)"("Value"=w176) -> ()  [unwired: 2 in, 2 out]
        n185 = property on="Station 11" class="Bool (strict)"("Value"=w176) -> ()  [unwired: 2 in, 2 out]
        n186 = property on="Station 12" class="Bool (strict)"("Value"=w176) -> ()  [unwired: 2 in, 2 out]
        n187 = property on="Station 13" class="Bool (strict)"("Value"=w176) -> ()  [unwired: 2 in, 2 out]
        n188 = property on="Station 14" class="Bool (strict)"("Value"=w176) -> ()  [unwired: 2 in, 2 out]
        n189 = property on="Station 15" class="Bool (strict)"("Value"=w176) -> ()  [unwired: 2 in, 2 out]
        n190 = property on="Station 16" class="Bool (strict)"("Value"=w176) -> ()  [unwired: 2 in, 2 out]
        n191 = property on="Station 17" class="Bool (strict)"("Value"=w176) -> ()  [unwired: 2 in, 2 out]
        n192 = property on="Station 18" class="Bool (strict)"("Value"=w176) -> ()  [unwired: 2 in, 2 out]
        n193 = property on="Station 19" class="Bool (strict)"("Value"=w176) -> ()  [unwired: 2 in, 2 out]
        n194 = property on="Station 20" class="Bool (strict)"("Value"=w176) -> ()  [unwired: 2 in, 2 out]
        n195 = property on="Station 21" class="Bool (strict)"("Value"=w176) -> ()  [unwired: 2 in, 2 out]
        n196 = property on="Select All" class="Bool (strict)"("DisabledEnum"=T1."Enabled" ("Disabled")) -> ()  [unwired: 2 in, 2 out]
        n197 = property on="Station 22" class="Bool (strict)"("Value"=w176) -> ()  [unwired: 2 in, 2 out]
        n198 = property on="Station 23" class="Bool (strict)"("Value"=w176) -> ()  [unwired: 2 in, 2 out]
        n199 = property on="Station 24" class="Bool (strict)"("Value"=w176) -> ()  [unwired: 2 in, 2 out]
        n200 = property on="Select All 1-4" class="Bool (strict)"("Value"=w176) -> ()  [unwired: 2 in, 2 out]
        n201 = property on="Select All 5-8" class="Bool (strict)"("Value"=w176) -> ()  [unwired: 2 in, 2 out]
        n202 = property on="Select All 9-12" class="Bool (strict)"("Value"=w176) -> ()  [unwired: 2 in, 2 out]
        n203 = property on="Select All 21-24" class="Bool (strict)"("Value"=w176) -> ()  [unwired: 2 in, 2 out]
        n204 = property on="Select All 13-16" class="Bool (strict)"("Value"=w176) -> ()  [unwired: 2 in, 2 out]
        n205 = property on="Select All 17-20" class="Bool (strict)"("Value"=w176) -> ()  [unwired: 2 in, 2 out]
        n206 = call "HCC Get Application Directory.vi"("Error In"=w171) -> ("Error Out"=w172:errorcluster, "Software Update Directory"=w167:path)  [unwired: 5 in, 4 out]
        "Main Directory" <- w167
        n207 = call "Software Update HCC Get Board IDs and Locations.vi"("Debug"=FALSE, "Error In"=w172, "Newfi Exe Folder Path"=w167) -> ("Error Out"=w170:errorcluster, "All Station Labels"=w177:string[])  [unwired: 5 in, 2 out]
        n208 = call <vilib>:"Add State(s) to Queue__jki_lib_state_machine.vi"("State(s) in (\"\")"=w181) -> ("States Out"=w180:string)  [unwired: 14 in]
        n209 = for {
          tunnel: w177 -> [w182] mode=indexing
          i -> [w183]
          n210 = case shown="23" w183 {
            tunnel: w182 -> [w186 w189 w192 w195 w197 w201 w204 w207 w210 w213 w216 w219 w222 w225 w228 w231 w234 w237 w240 w243 w246 w249 w252 w255]
            frame 0, Default {
              n211 = Build Array(w186) -> (w185:string[])
              n212 = property on="Station 1" class="Bool (strict)"("BoolText.Visible"=TRUE ("Boolean Text.Visible"), "Strings [4]"=w185) -> ()  [unwired: 2 in, 2 out]
            }
            frame 1 {
              n213 = Build Array(w189) -> (w188:string[])
              n214 = property on="Station 2" class="Bool (strict)"("BoolText.Visible"=TRUE ("Boolean Text.Visible"), "Strings [4]"=w188) -> ()  [unwired: 2 in, 2 out]
            }
            frame 2 {
              n215 = Build Array(w192) -> (w191:string[])
              n216 = property on="Station 3" class="Bool (strict)"("BoolText.Visible"=TRUE ("Boolean Text.Visible"), "Strings [4]"=w191) -> ()  [unwired: 2 in, 2 out]
            }
            frame 3 {
              n217 = Build Array(w195) -> (w194:string[])
              n218 = property on="Station 4" class="Bool (strict)"("BoolText.Visible"=TRUE ("Boolean Text.Visible"), "Strings [4]"=w194) -> ()  [unwired: 2 in, 2 out]
            }
            frame 4 {
              n219 = Build Array(w197) -> (w196:string[])
              n220 = property on="Station 5" class="Bool (strict)"("BoolText.Visible"=TRUE ("Boolean Text.Visible"), "Strings [4]"=w196) -> ()  [unwired: 2 in, 2 out]
            }
            frame 5 {
              n221 = Build Array(w201) -> (w200:string[])
              n222 = property on="Station 6" class="Bool (strict)"("BoolText.Visible"=TRUE ("Boolean Text.Visible"), "Strings [4]"=w200) -> ()  [unwired: 2 in, 2 out]
            }
            frame 6 {
              n223 = Build Array(w204) -> (w203:string[])
              n224 = property on="Station 7" class="Bool (strict)"("BoolText.Visible"=TRUE ("Boolean Text.Visible"), "Strings [4]"=w203) -> ()  [unwired: 2 in, 2 out]
            }
            frame 7 {
              n225 = Build Array(w207) -> (w206:string[])
              n226 = property on="Station 8" class="Bool (strict)"("BoolText.Visible"=TRUE ("Boolean Text.Visible"), "Strings [4]"=w206) -> ()  [unwired: 2 in, 2 out]
            }
            frame 8 {
              n227 = Build Array(w210) -> (w209:string[])
              n228 = property on="Station 9" class="Bool (strict)"("BoolText.Visible"=TRUE ("Boolean Text.Visible"), "Strings [4]"=w209) -> ()  [unwired: 2 in, 2 out]
            }
            frame 9 {
              n229 = Build Array(w213) -> (w212:string[])
              n230 = property on="Station 10" class="Bool (strict)"("BoolText.Visible"=TRUE ("Boolean Text.Visible"), "Strings [4]"=w212) -> ()  [unwired: 2 in, 2 out]
            }
            frame 10 {
              n231 = Build Array(w216) -> (w215:string[])
              n232 = property on="Station 11" class="Bool (strict)"("BoolText.Visible"=TRUE ("Boolean Text.Visible"), "Strings [4]"=w215) -> ()  [unwired: 2 in, 2 out]
            }
            frame 11 {
              n233 = Build Array(w219) -> (w218:string[])
              n234 = property on="Station 12" class="Bool (strict)"("BoolText.Visible"=TRUE ("Boolean Text.Visible"), "Strings [4]"=w218) -> ()  [unwired: 2 in, 2 out]
            }
            frame 12 {
              n235 = Build Array(w222) -> (w221:string[])
              n236 = property on="Station 13" class="Bool (strict)"("BoolText.Visible"=TRUE ("Boolean Text.Visible"), "Strings [4]"=w221) -> ()  [unwired: 2 in, 2 out]
            }
            frame 13 {
              n237 = Build Array(w225) -> (w224:string[])
              n238 = property on="Station 14" class="Bool (strict)"("BoolText.Visible"=TRUE ("Boolean Text.Visible"), "Strings [4]"=w224) -> ()  [unwired: 2 in, 2 out]
            }
            frame 14 {
              n239 = Build Array(w228) -> (w227:string[])
              n240 = property on="Station 15" class="Bool (strict)"("BoolText.Visible"=TRUE ("Boolean Text.Visible"), "Strings [4]"=w227) -> ()  [unwired: 2 in, 2 out]
            }
            frame 15 {
              n241 = Build Array(w231) -> (w230:string[])
              n242 = property on="Station 16" class="Bool (strict)"("BoolText.Visible"=TRUE ("Boolean Text.Visible"), "Strings [4]"=w230) -> ()  [unwired: 2 in, 2 out]
            }
            frame 16 {
              n243 = Build Array(w234) -> (w233:string[])
              n244 = property on="Station 17" class="Bool (strict)"("BoolText.Visible"=TRUE ("Boolean Text.Visible"), "Strings [4]"=w233) -> ()  [unwired: 2 in, 2 out]
            }
            frame 17 {
              n245 = Build Array(w237) -> (w236:string[])
              n246 = property on="Station 18" class="Bool (strict)"("BoolText.Visible"=TRUE ("Boolean Text.Visible"), "Strings [4]"=w236) -> ()  [unwired: 2 in, 2 out]
            }
            frame 18 {
              n247 = Build Array(w240) -> (w239:string[])
              n248 = property on="Station 19" class="Bool (strict)"("BoolText.Visible"=TRUE ("Boolean Text.Visible"), "Strings [4]"=w239) -> ()  [unwired: 2 in, 2 out]
            }
            frame 19 {
              n249 = Build Array(w243) -> (w242:string[])
              n250 = property on="Station 20" class="Bool (strict)"("BoolText.Visible"=TRUE ("Boolean Text.Visible"), "Strings [4]"=w242) -> ()  [unwired: 2 in, 2 out]
            }
            frame 20 {
              n251 = Build Array(w246) -> (w245:string[])
              n252 = property on="Station 21" class="Bool (strict)"("BoolText.Visible"=TRUE ("Boolean Text.Visible"), "Strings [4]"=w245) -> ()  [unwired: 2 in, 2 out]
            }
            frame 21 {
              n253 = Build Array(w249) -> (w248:string[])
              n254 = property on="Station 22" class="Bool (strict)"("BoolText.Visible"=TRUE ("Boolean Text.Visible"), "Strings [4]"=w248) -> ()  [unwired: 2 in, 2 out]
            }
            frame 22 {
              n255 = Build Array(w252) -> (w251:string[])
              n256 = property on="Station 23" class="Bool (strict)"("BoolText.Visible"=TRUE ("Boolean Text.Visible"), "Strings [4]"=w251) -> ()  [unwired: 2 in, 2 out]
            }
            frame 23 {
              n257 = Build Array(w255) -> (w254:string[])
              n258 = property on="Station 24" class="Bool (strict)"("BoolText.Visible"=TRUE ("Boolean Text.Visible"), "Strings [4]"=w254) -> ()  [unwired: 2 in, 2 out]
            }
          }
        }
        n259 = call "UTILITY Find Newfi Device.vi"() -> ("Array of Newfi Devices"=→"Board ID's":string[], "Number of Newfi's"=→"Number of Newfi's":i32)  [unwired: 8 in, 2 out]
        n260 = Bundle By Name(cluster=w169, "Base Newfi Exe Folder Path"=w167) -> (w168:T5)
      }
      frame "UI: Cursor Set" {
        # "Argument"
        # "Set and Unset Cursor Busy.\n(Usage: \"UI: Cursor Set >> Busy|Idle\")"
        n261 = case shown="\"Idle\", Default" w256 {
          tunnel: w258 -> [w263 w265]
          tunnel: [w262 w264] -> w257
          frame "Idle", Default {
            n262 = call <vilib>:"Unset Busy.vi"("error in (no error)"=w263) -> ("error out"=w262:errorcluster)  [unwired: 10 in]
          }
          frame "Busy" {
            n263 = call <vilib>:"Set Busy.vi"("error in (no error)"=w265) -> ("error out"=w264:errorcluster)  [unwired: 9 in, 1 out]
          }
        }
        n264 = call <vilib>:"Add State(s) to Queue__jki_lib_state_machine.vi"("State(s) in (\"\")"=w261) -> ("States Out"=w260:string)  [unwired: 14 in]
      }
      frame "UI: Front Panel State" {
        # "Argument"
        # "Set Front Panel Open or Closed\n(Usage: \"UI: Front Panel State >> Open|Close\")"
        n265 = Unbundle By Name(w268) -> ("Core.Current VI Reference"=w267:refnum<vi>)
        n266 = case shown="\"Open\", Default" w266 {
          tunnel: w270 -> [w276 w289]
          tunnel: [w278 w290] -> w269
          tunnel: w267 -> [w277 w287]
          frame "Open", Default {
            n267 = property class="VI"(reference=w277, error in=w276) -> (reference out=w274:refnum<vi>, error out=w275:errorcluster, "Front Panel.Open"=w273:bool)
            n268 = case shown="False" w273 {
              tunnel: [w281 w284] -> w278
              tunnel: w275 -> [w280 w284]
              tunnel: w274 -> [w279 _]
              frame False {
                n269 = invoke class="VI" method="FP.Open"(reference=w279, error in=w280, "Activate"=TRUE, "State"=T4."Standard") -> (error out=w281:errorcluster)  [unwired: 1 in, 4 out]
              }
              frame True {
              }
            }
          }
          frame "Close" {
            n270 = property class="VI"(reference=w287, error in=w289) -> (reference out=w286:refnum<vi>, error out=w288:errorcluster, "Front Panel.Open"=w285:bool)
            n271 = case shown="True" w285 {
              tunnel: [w291 w294] -> w290
              tunnel: w288 -> [w291 w293]
              tunnel: w286 -> [_ w292]
              frame False {
              }
              frame True {
                n272 = invoke class="VI" method="FP.Close"(reference=w292, error in=w293) -> (error out=w294:errorcluster)  [unwired: 1 in, 2 out]
              }
            }
          }
        }
        n273 = call <vilib>:"Add State(s) to Queue__jki_lib_state_machine.vi"("State(s) in (\"\")"=w272) -> ("States Out"=w271:string)  [unwired: 14 in]
      }
      frame "---------- Macro ----------" {
        # "Do not put any code in this frame.\n(It is a separator no-op. You can make a copy of this frame to create a new Macro frame)"
        n274 = call <vilib>:"Add State(s) to Queue__jki_lib_state_machine.vi"("State(s) in (\"\")"=w298) -> ("States Out"=w297:string)  [unwired: 14 in]
      }
      frame "Macro: Initialize" {
        w299 = "Data: Initialize\nInitialize Core Data\nUI: Initialize\nUI: Front Panel State >> Open"  # Data: Initialize Initialize Core Data UI: Initialize UI: Front Panel State >> Open
        n275 = call <vilib>:"Add State(s) to Queue__jki_lib_state_machine.vi"("State(s) in Front (\"\")"=w299, "State(s) in (\"\")"=w303) -> ("States Out"=w302:string)  [unwired: 13 in]
      }
      frame "Macro: Exit" {
        # "Exit Macro\n(This is called once, when the VI exits)"
        n276 = Unbundle By Name(w311) -> ("Core.Close Panel on Exit?"=w310:bool)
        n277 = local write "Status String"("Complete..." ("Status String")) -> ()
        n278 = Select(t="UI: Front Panel State >> Close", s=w310, f="") -> (s? t:f=w307:string)
        n279 = call <vilib>:"Add State(s) to Queue__jki_lib_state_machine.vi"("State(s) in (\"\")"=w307, "State(s) at Back (\"\")"="Data: Cleanup\nExit") -> ("States Out"=w305:string)  [unwired: 13 in]
        n280 = call <vilib>:"Add State(s) to Queue__jki_lib_state_machine.vi"("State(s) in Front (\"\")"=w305, "State(s) in (\"\")"=w314) -> ("States Out"=w313:string)  [unwired: 13 in]
      }
      frame "---------- New Category ----------" {
        # "Template Separator\n(You can make a copy of, or modify, this frame)"
        n281 = call <vilib>:"Add State(s) to Queue__jki_lib_state_machine.vi"("State(s) in (\"\")"=w318) -> ("States Out"=w317:string)  [unwired: 14 in]
      }
      frame "Station Update List" {
        n282 = Build Array("Station 1", "Station 2", "Station 3", "Station 4", "Station 5", "Station 6", "Station 7", "Station 8", "Station 9", "Station 10", "Station 11", "Station 12", "Station 13", "Station 14", "Station 15", "Station 16", "Station 17", "Station 18", "Station 19", "Station 20", "Station 21", "Station 22", "Station 23", "Station 24") -> (w351:bool[])
        n283 = call "Software Update HCC Populate Update File List.vi"("Error In"=w320, "Stations to Update"=w351) -> ("Error Out"=w319:errorcluster, "Update List"=w323:i32[])  [unwired: 8 in]
        n284 = Array Size(array=w323) -> (size(s)=w322:i32)
        n285 = Bundle By Name(cluster=w350, "Update Files (Option 1-24)"=w323) -> (w349:T5)
        n286 = Equal To 0?(x=w322) -> (x = 0?=w321:bool)
        n287 = case shown="True" w321 {
          frame False {
          }
          frame True {
            n288 = One Button Dialog(message="Select A Station") -> ()  [unwired: 1 in, 1 out]
          }
        }
        n289 = call <vilib>:"Add State(s) to Queue__jki_lib_state_machine.vi"("State(s) in (\"\")"=w353) -> ("States Out"=w352:string)  [unwired: 14 in]
        "Status String" <- "Compiling Update List..." ("Status String")
      }
      frame "Build Paths" {
        n290 = Unbundle By Name(w360) -> ("Base Newfi Exe Folder Path"=w355:path, "Update Files (Option 1-24)"=w361:i32[])
        n291 = call "Software Update HCC Build EXE Locations.vi"("Error In"=w357, "Update Files (Option 1-24)"=w361, "Newfi Exe Folder Path"=w355) -> ("Error Out"=w356:errorcluster, "Path Build List (Folder Locations)"=w358:path[])  [unwired: 7 in]
        n292 = Bundle By Name(cluster=w360, "Path Build List"=w358) -> (w359:T5)
        n293 = call <vilib>:"Add State(s) to Queue__jki_lib_state_machine.vi"("State(s) in (\"\")"=w363) -> ("States Out"=w362:string)  [unwired: 14 in]
      }
      frame "Update Test Software" {
        n294 = Unbundle By Name(w374) -> ("Path Build List"=w376:path[], "Base Newfi Exe Folder Path"=w367:path, "Update Files (Option 1-24)"=w366:i32[])
        n295 = control-ref of="% Complete"() -> (w373:refnum<vi>)
        n296 = call "Software Update HCC Update Software.vi"("% Complete"=w373, "Path Build List Sub"=w376, "Error In"=w365, "Update Files (Option 1-24) Sub"=w366, "Newfi Exe Folder Path"=w367, "New Software Location"="New Software Location") -> ("Error Out"=w364:errorcluster)  [unwired: 5 in]
        n297 = Strip Path(path="New Software Location") -> (name=w370:string)  [unwired: 1 out]
        n298 = call <vilib>:"Add State(s) to Queue__jki_lib_state_machine.vi"("State(s) in (\"\")"=w378) -> ("States Out"=w377:string)  [unwired: 14 in]
        n299 = call <vilib>:"Space Constant.vi"() -> ("String"=w371:string)
        n300 = Concatenate Strings("Downloading" ("string"), w371, w370, "..." ("string")) -> (w369:string)
        n301 = local write "Status String"(w369) -> ()
      }
      frame "Final Update" {
        n302 = local write "Newfi"(FALSE ("Newfi")) -> ()
        n303 = local write "% Complete"(u8 100 ("% Complete")) -> ()
        n304 = property on="Newfi" class="Bool (strict)"("DisabledEnum"=T1."Enabled" ("Disabled")) -> ()  [unwired: 2 in, 2 out]
        n305 = local write "Status String"("Complete...." ("Status String")) -> ()
        n306 = call <vilib>:"Add State(s) to Queue__jki_lib_state_machine.vi"("State(s) in (\"\")"=w386) -> ("States Out"=w385:string)  [unwired: 14 in]
      }
    }
    n307 = case shown="True" "Debug" {
      tunnel: w12 -> [w23 w26]
      tunnel: w10 -> [_ w25]
      tunnel: [w23 w24] -> w9
      frame False {
      }
      frame True {
        n308 = Build Array (concatenate)(w26, w25) -> (w24:string[])
        "Debug Array" <- w24
      }
    }
  }
